vi "Vowel-Initialize.vi"(0 "Vowel In":T1, 11 "error in (no error)":errorcluster) -> (4 "Vowel Out":T1, 15 "error out":errorcluster)   [LabVIEW 2020]
uses:
  XControls/Waveform XControls/Vowel/Vowel.Properties.ctl
  XControls/Waveform XControls/Vowel/Vowel.xctl
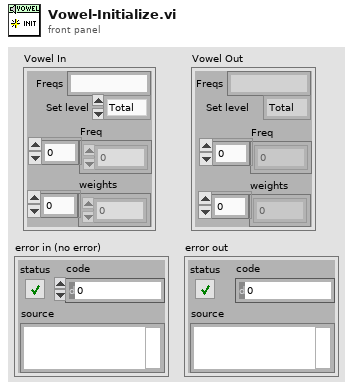
[diagram p1: front panel]
types:
  T1 = typedef "Vowel.xctl/Vowel.Properties.ctl" = cluster{"Freqs":string, "Set level":enum16{"Total", "Per component"}, "Freq":dbl[], "weights":dbl[]}
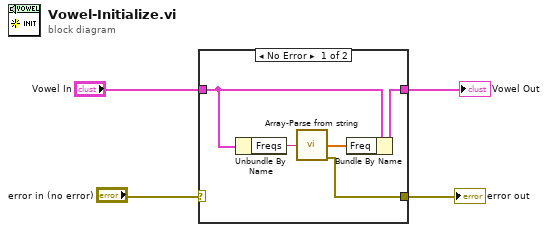
[diagram p0: block diagram]
diagram:
  n1 = case shown="No Error" "error in (no error)" {
    selector: "error in (no error)" -> [_ w11]
    tunnel: "Vowel In" -> [w8 w10]
    tunnel: [w9 w11] -> w3
    tunnel: [w6 w10] -> w4
    frame No Error {
      n2 = Unbundle By Name(w8) -> ("Freqs"=w7:string)
      n3 = call "Array-Parse from string.vi"("String"=w7) -> ("Array"=w5:dbl[], "error out"=w9:errorcluster)  [unwired: 13 in]
      n4 = Bundle By Name(cluster=w8, "Freq"=w5) -> (w6:T1)
    }
    frame Error {
    }
  }
  "Vowel Out" <- w4
  "error out" <- w3
